vi "Turret_Execute.vi"() -> ()   [LabVIEW 2019]
uses:
  <vilib>/Rock Robotics/WPI/ThirdParty/Phoenix-LabVIEW/Motor Controller/Controls/CTRE_Phoenix_MotorControl_ControlMode.ctl
  Turret_Globals.vi
  Sensor_Values.vi
panel:
  in  "Kp position":dbl
  in  "Kp Aim":dbl=0.08
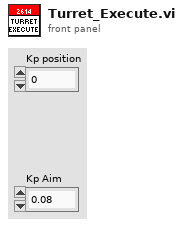
[diagram p1: front panel]
types:
  T1 = typedef "WPI_MotorControlDeviceRef.ctl" = cluster{"DeviceStatus":errorcluster, "Type":T2, "PWM":cluster{"PWM Channel":T3, "DeadBand":T4}, "CAN":cluster{"Device Number":u8, "SetOutput VI Ref":variant, "GetOutput VI Ref":variant, "Enable VI Ref":variant, "Disable VI Ref":variant, "Data":variant}, "Invert":bool, "DIO PWM":cluster{"PWM \"Enable\" Channel":T3, "DIOChannel":T5, "PWM Rate":dbl}}
  T2 = typedef "WPI_MotorControlType.ctl" = enum16{"PWM", "CAN", "DIO PWM"}
  T3 = typedef "FPGA_DIOPWMChannel.ctl" = enum8{"PWM 0", "PWM 1", "PWM 2", "PWM 3", "PWM 4", "PWM 5", "PWM 6", "PWM 7", "PWM 8", "PWM 9", "PWM MXP 0", "PWM MXP 1", "PWM MXP 2", "PWM MXP 3", "PWM MXP 4", "PWM MXP 5", "PWM MXP 6", "PWM MXP 7", "PWM MXP 8", "PWM MXP 9", "Invalid"}
  T4 = typedef "WPI_PWMDeadband.ctl" = cluster{"Name":string, "maxPositivePwm":i32, "minPositivePwm":i32, "centerPwm":i32, "maxNegativePwm":i32, "minNegativePwm":i32, "angularRange":u16}
  T5 = typedef "FPGA_DIOChannel.ctl" = enum8{"DIO 0", "DIO 1", "DIO 2", "DIO 3", "DIO 4", "DIO 5", "DIO 6", "DIO 7", "DIO 8", "DIO 9", "DIO MXP 0", "DIO MXP 1", "DIO MXP 2", "DIO MXP 3", "DIO MXP 4", "DIO MXP 5", "DIO MXP 6", "DIO MXP 7", "DIO MXP 8", "DIO MXP 9", "DIO MXP 10", "DIO MXP 11", "DIO MXP 12", "DIO MXP 13", "DIO MXP 14", "DIO MXP 15", "SPI Port CS1", "SPI Port CS2", "SPI Port CS3", "SPI Port MISO", "SPI Port MOSI", "Invalid"}
  T6 = typedef "Turret_Cluster.ctl" = cluster{"Control_State":enum16{"Manual_PercentVoltage", "Manual_SpeedControl", "Auto_Targeting", "Position"}, "Spin_Power":dbl, "Flywheel_Power":dbl, "Going_To_Position":bool}
  T7 = enum16{"Manual_PercentVoltage", "Manual_SpeedControl", "Auto_Targeting", "Position"}
  T8 = typedef "CTRE_Phoenix_MotorControl_ControlMode.ctl" = u16
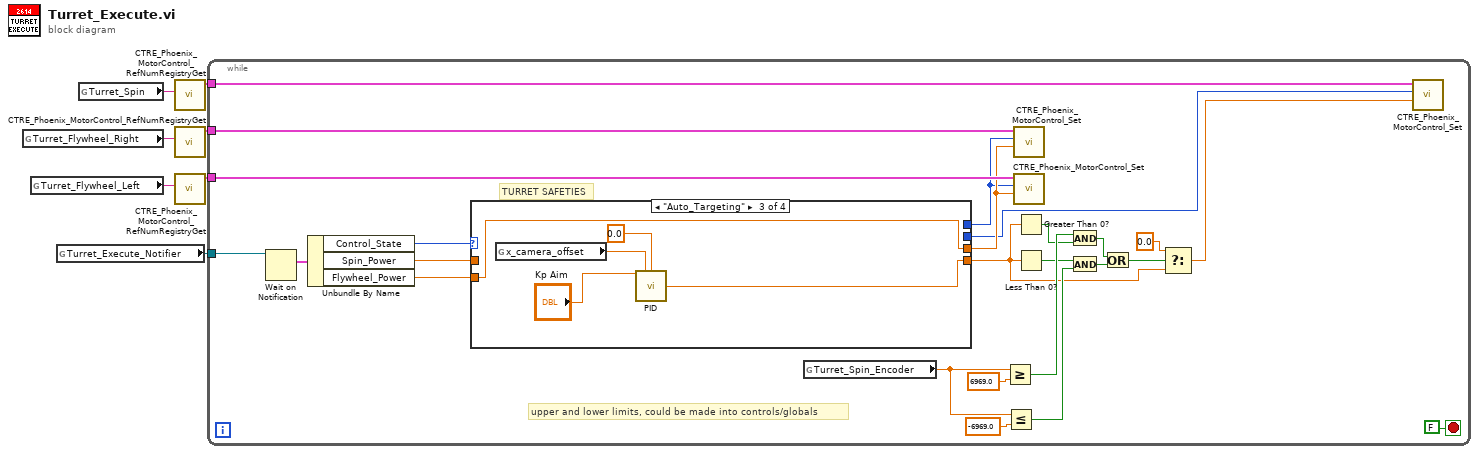
[diagram p0: block diagram]
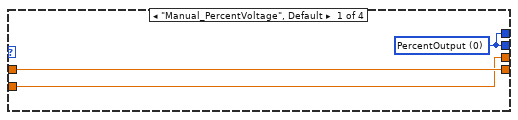
[diagram p2: hidden frame]
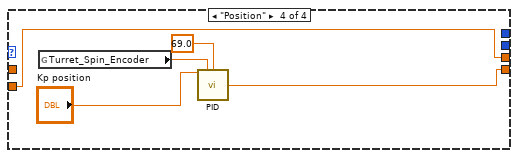
[diagram p4: hidden frame]
diagram:
  n1 = global read "Turret_Globals.vi" "Turret_Flywheel_Right"() -> (w6:string)
  n2 = global read "Turret_Globals.vi" "Turret_Flywheel_Left"() -> (w5:string)
  n3 = global read "Turret_Globals.vi" "Turret_Execute_Notifier"() -> (w7:refnum<notifier>)
  n4 = global read "Turret_Globals.vi" "Turret_Spin"() -> (w4:string)
  n5 = call <vilib>:"CTRE_Phoenix_MotorControl_RefNumRegistryGet.vi"("refnum name"=w4) -> ("PhoenixMotorControlDevRef"=w3:T1)  [unwired: 9 in, 1 out]
  n6 = call <vilib>:"CTRE_Phoenix_MotorControl_RefNumRegistryGet.vi"("refnum name"=w6) -> ("PhoenixMotorControlDevRef"=w1:T1)  [unwired: 9 in, 1 out]
  n7 = call <vilib>:"CTRE_Phoenix_MotorControl_RefNumRegistryGet.vi"("refnum name"=w5) -> ("PhoenixMotorControlDevRef"=w2:T1)  [unwired: 9 in, 1 out]
  n8 = while {
    tunnel: w7 -> [w31]
    tunnel: w3 -> [w28]
    tunnel: w2 -> [w27]
    tunnel: w1 -> [w26]
    stop <- FALSE stop-if-true
    # "upper and lower limits, could be made into controls/globals"
    # "TURRET SAFETIES"
    n9 = Wait on Notification(notifier=w31) -> (notification=w30:T6)  [unwired: 3 in, 3 out]
    n10 = Unbundle By Name(w30) -> ("Control_State"=w29:T7, "Spin_Power"=w25:dbl, "Flywheel_Power"=w24:dbl)
    n11 = case shown="\"Auto_Targeting\"" w29 {
      tunnel: w25 -> [w35 _ _ _]
      tunnel: w24 -> [w34 _ w39 w42]
      tunnel: [w35 _ w38 w41] -> w12
      tunnel: [w34 _ w39 w42] -> w23
      tunnel: [w33 _ _ _] -> w22
      tunnel: [w33 _ _ _] -> w21
      frame "Manual_PercentVoltage", Default {
        w33 = T8 0 items=["PercentOutput"=0, "Position"=1, "Velocity"=2, "Current"=3, "Follower"=5, "MotionProfile"=6, "MotionMagic"=7, "MotionProfileArc"=10, "Disabled"=15] ("Control Mode")
      }
      frame "Manual_SpeedControl" {
        # "need encoders for speed control"
      }
      frame "Auto_Targeting" {
        n12 = global read "Sensor_Values.vi" "x_camera_offset"() -> (w36:dbl)
        n13 = call "PID.vi"("Kp"="Kp Aim", "Process Variable"=w36, "Goal"=0.0) -> ("Command"=w38:dbl)  [unwired: 10 in, 2 out]
      }
      frame "Position" {
        n14 = global read "Sensor_Values.vi" "Turret_Spin_Encoder"() -> (w45:dbl)
        n15 = call "PID.vi"("Kp"="Kp position", "Process Variable"=w45, "Goal"=69.0) -> ("Command"=w41:dbl)  [unwired: 10 in, 2 out]
      }
    }
    n16 = global read "Sensor_Values.vi" "Turret_Spin_Encoder"() -> (w10:dbl)
    n17 = Greater Or Equal?(x=w10, y=6969.0) -> (x >= y?=w20:bool)
    n18 = Less Or Equal?(x=w10, y=-6969.0) -> (x <= y?=w18:bool)
    n19 = call <vilib>:"CTRE_Phoenix_MotorControl_Set.vi"("Output"=w23, "Control Mode"=w21, "PhoenixMotorControlDevRef"=w26) -> ()  [unwired: 7 in, 2 out]
    n20 = call <vilib>:"CTRE_Phoenix_MotorControl_Set.vi"("Output"=w23, "Control Mode"=w21, "PhoenixMotorControlDevRef"=w27) -> ()  [unwired: 7 in, 2 out]
    n21 = Greater Than 0?(x=w12) -> (x > 0?=w19:bool)
    n22 = Less Than 0?(x=w12) -> (x < 0?=w17:bool)
    n23 = And(x=w20, y=w19) -> (x .and. y?=w15:bool)
    n24 = And(x=w17, y=w18) -> (x .and. y?=w16:bool)
    n25 = Or(x=w15, y=w16) -> (x .or. y?=w14:bool)
    n26 = Select(t=0.0, s=w14, f=w12) -> (s? t:f=w8:dbl)
    n27 = call <vilib>:"CTRE_Phoenix_MotorControl_Set.vi"("Output"=w8, "Control Mode"=w22, "PhoenixMotorControlDevRef"=w28) -> ()  [unwired: 7 in, 2 out]
  }
